vi "Global_CMD_CMD_Data In.vi"() -> ()   [LabVIEW 2023, in "2023-Auto_CMD.lvlib"]
uses:
  2023-Auto_CMD.lvlib
  Cluster_CMD_CMD_Data.ctl
  Shared Code/TypeDefs/ENUM_AutoSelect.ctl
panel:
  in  "CMD_CMD_2024-Auto_Data":T1
  # "The Names of the Data items in the Global Variable MUST describe who the Single Writer is\nFor Command Globals the Commander(CMD) represents Teleop or Autonomous or other command loop.\nThe naming convention for a Command for a Command Global is:   \n\nCMD_CMD_LibName_Data Name\n\nExample:\nCMD_CMD_BallShooter_Data\nCMD_CMD_ProgramedMotion1_Data"
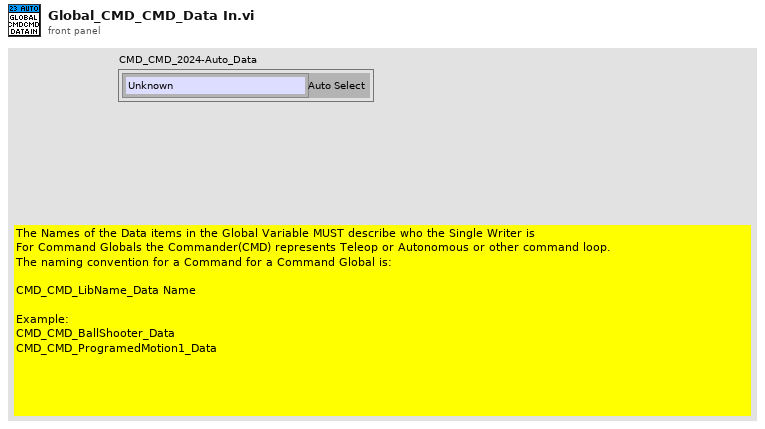
[diagram p1: front panel]
types:
  T1 = typedef "2023-Auto_CMD.lvlib/Cluster_CMD_CMD_Data.ctl" = cluster{"Auto Select":T2}
  T2 = typedef "ENUM_AutoSelect.ctl" = enum16{"Unknown", "Shoot and Drive Center", "Shoot and Drive SpeakerLeft", "Shoot and Drive SpeakerRight"}
diagram:
